vi "GetVIFromSubPanelByPathArray.vi"(0 "VI Reference in":refnum<vi>, 5 "SubPanel Path":string[](array[string]), 11 "error in (no error)":errorcluster) -> (4 "VI Reference out":refnum<vi>, 6 "SubPanel VI Reference":refnum<vi>, 15 "error out":errorcluster)   [LabVIEW 2016]
doc: "This VI gives the reference of the inserted VI in the SubPanel.\n\nThe SubPanel path input can be given in successive index of the array."
uses:
  ControlAction/GetSubPanelVI/GetSubPanelVI.lvclass
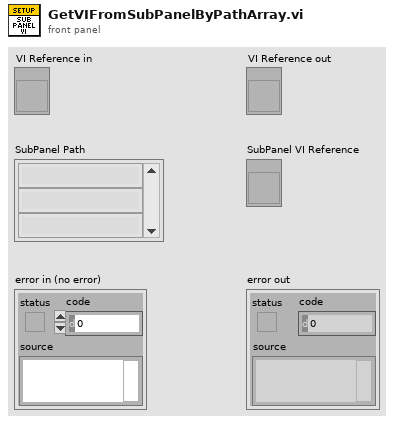
[diagram p1: front panel]
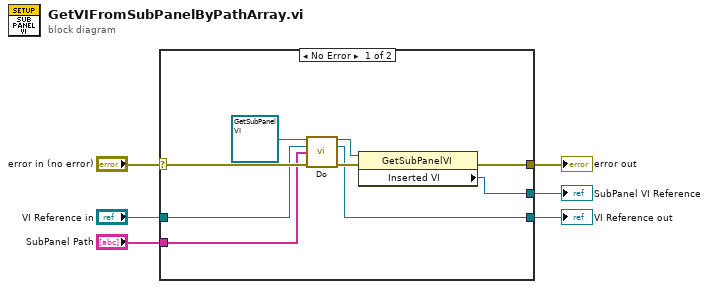
[diagram p0: block diagram]
diagram:
  n1 = case shown="No Error" "error in (no error)" {
    selector: "error in (no error)" -> [w15 w17]
    tunnel: [w12 w17] -> w5
    tunnel: "SubPanel Path" -> [w13 _]
    tunnel: [w9 _] -> w3
    tunnel: "VI Reference in" -> [w8 w16]
    tunnel: [w7 w16] -> w1
    frame No Error {
      n2 = call-dynamic "Do.vi"("ControlDoBase in"=refnum<class "GetSubPanelVI.lvclass"> refnum ("GetSubPanelVI"), "VI Reference in"=w8, "Control Path"=w13, "error in"=w15) -> ("ControlDoBase out"=w10:refnum<class "GetSubPanelVI.lvclass">, "VI Reference out"=w7:refnum<vi>, "error out"=w14:errorcluster)  [unwired: 9 in]
      n3 = property class="GetSubPanelVI"(reference=w10, error in=w14) -> (error out=w12:errorcluster, "Inserted VI"=w9:refnum<vi>)  [unwired: 1 out]
    }
    frame Error {
    }
  }
  "error out" <- w5
  "SubPanel VI Reference" <- w3
  "VI Reference out" <- w1
